vi "PhotoName.vi"(1 "String":string, 2 "PhotoPath":path) -> (0 "path":path)   [LabVIEW 2016, in "CCD monitor.lvlib" / "CCD monitor.lvclass"]
uses:
  <userlib>/Common Components/Hardware/Abstract System/Monitor/CCD monitor.lvclass
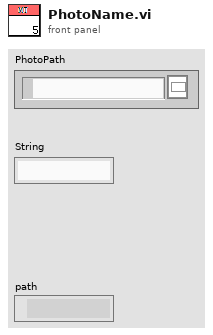
[diagram p1: front panel]
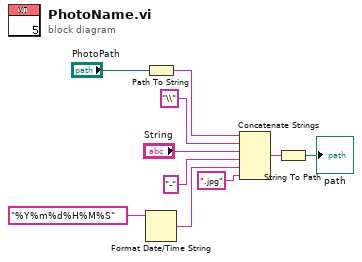
[diagram p0: block diagram]
diagram:
  n1 = Path To String(path="PhotoPath") -> (string=w9:string)
  n2 = Format Date/Time String(time format string (%c)="%Y%m%d%H%M%S") -> (date/time string=w1:string)  [unwired: 2 in]
  n3 = Concatenate Strings(w9, "\\", "String", "-" ("string"), w1, ".jpg") -> (w4:string)
  n4 = String To Path(string=w4) -> (path=→"path":path)
